vi "Panel.vi"(11 "SequenceViewPanel in":refnum<class "SequenceViewPanel.lvclass">) -> ()   [LabVIEW 2020, in "TSnax UI.lvlib" / "SequenceViewPanel.lvclass"]
uses:
  SequenceViewPanel.lvclass
  C:/Program Files (x86)/National Instruments/LabVIEW 2020/vi.lib/IlluminatedG/IG OOPanel/OOPanel/Panel/Panel.lvclass
  <vilib>/IlluminatedG/IG OOPanel/OOPanel/Panel/Basic UI State.ctl
  <vilib>/IlluminatedG/IG OOPanel/OOPanel/Panel/Panel Events.ctl
  <vilib>/IlluminatedG/IG OOPanel/OOPanel/Panel/Visbility Event Data.ctl
  <vilib>/IlluminatedG/IG OOPanel/OOPanel/Panel/Visibility State.ctl
  <vilib>/IlluminatedG/IG OOPanel/OOPanel/Panel/Close Reason.ctl
  Incoming Events.ctl
  Set SequenceFile Request.ctl
  TSnax/SequenceFile/SequenceFile.lvclass
  C:/dev/illuminated-g/tsnax/TSnax/PropertyObject/PropertyObject.lvclass
  SequenceViewPanel.lvclass/SequenceViewPanel.ctl
  TSnax/PropertyObject/PropertyObject.lvclass/PropertyObject.ctl
  TSnax/PropertyObject/PropertyObject Ref.vi
  TSnax/PropertyObject/PropertyObject.lvclass
  <vilib>/IlluminatedG/IG OOPanel/OOPanel/Panel/Panel.lvclass
  <vilib>/IlluminatedG/IG OOPanel/OOPanel/OOPanel.lvlib
  C:/dev/illuminated-g/tsnax/TSnax UI/SequenceViewPanel/SequenceViewPanel.lvclass
  Set SequenceFile Response.ctl
  C:/dev/illuminated-g/tsnax/TSnax/PropertyObjectFile/PropertyObjectFile.lvclass
  C:/dev/illuminated-g/tsnax/TSnax/SequenceFile/SequenceFile.lvclass
panel:
  out "Markers":picture
  in  "Steps":string(tree)
  in  "Sequences":string(tree)
  in  "Variables":string(tree)
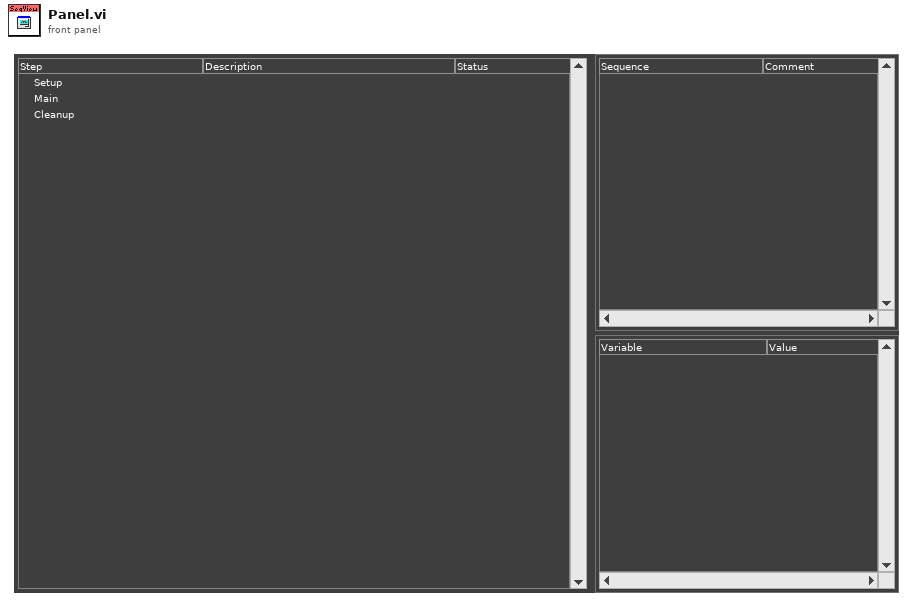
[diagram p1: front panel]
types:
  T1 = typedef "OOPanel.lvlib/Panel.lvclass/Basic UI State.ctl" = enum16{"Init", "Run", "Close"}
  T2 = typedef "TSnax UI.lvlib/SequenceViewPanel.lvclass/Set SequenceFile Response.ctl" = cluster{"Error":errorcluster}
  T3 = typedef "TSnax UI.lvlib/SequenceViewPanel.lvclass/Incoming Events.ctl" = cluster{"Set SequenceFile":refnum<user-event>}
  T4 = typedef "OOPanel.lvlib/Panel.lvclass/Panel Events.ctl" = cluster{"Visbility":refnum<user-event>, "Close":refnum<user-event>}
  T5 = cluster{"Panel":refnum<event-registration>, "Refresh Markers Reg":refnum<event-registration>}
  T6 = typedef "OOPanel.lvlib/Visibility State.ctl" = enum16{"Idle", "Closed", "Hidden", "Visible", "Subpanel"}
  T7 = typedef "LVRectTypeDef.ctl" = cluster{"Left":i16, "Top":i16, "Right":i16, "Bottom":i16}
  T8 = typedef "LVBoundsTypeDef.ctl" = cluster{"Width":u32, "Height":u32}
  T9 = typedef "LVPoint32TypeDef.ctl" = cluster{"Horizontal":i32, "Vertical":i32}
  T10 = typedef "TSnax UI.lvlib/SequenceViewPanel.lvclass/Ref Data.ctl" = cluster{"Insert Index":i32, "SequenceFile":refnum<class "SequenceFile.lvclass">}
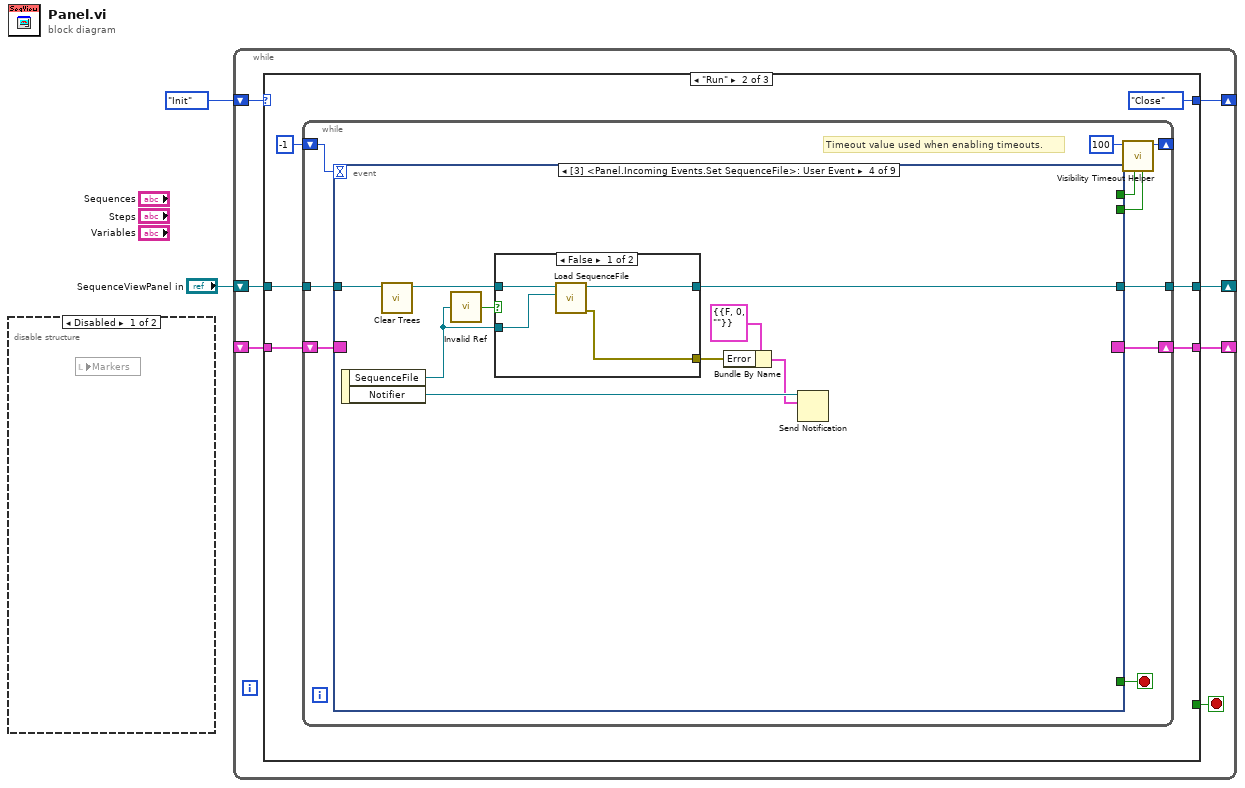
[diagram p0: block diagram]
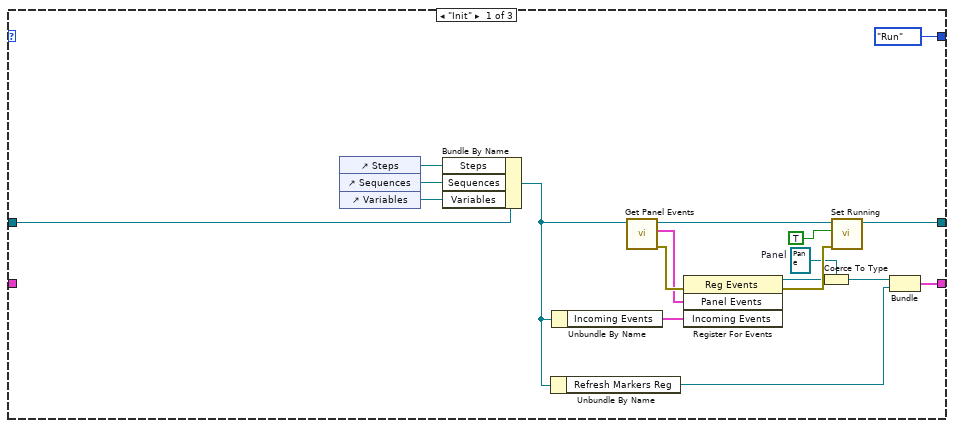
[diagram p3: hidden frame]
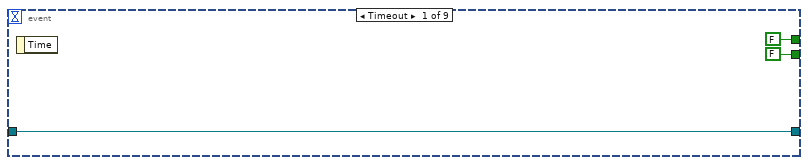
[diagram p4: hidden frame]
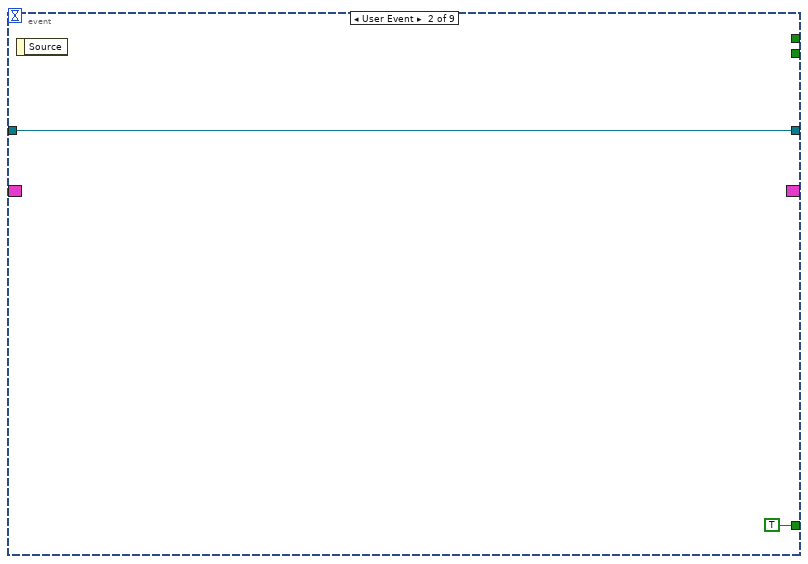
[diagram p5: hidden frame]
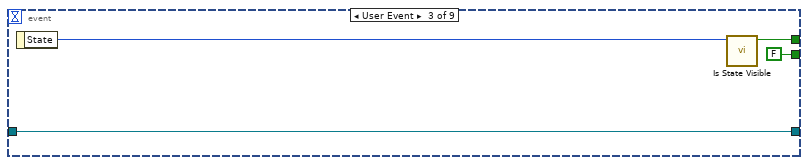
[diagram p6: hidden frame]
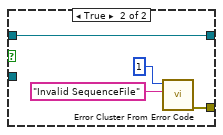
[diagram p7: hidden frame]
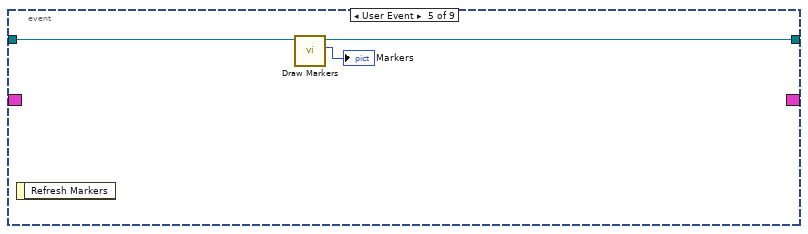
[diagram p8: hidden frame]
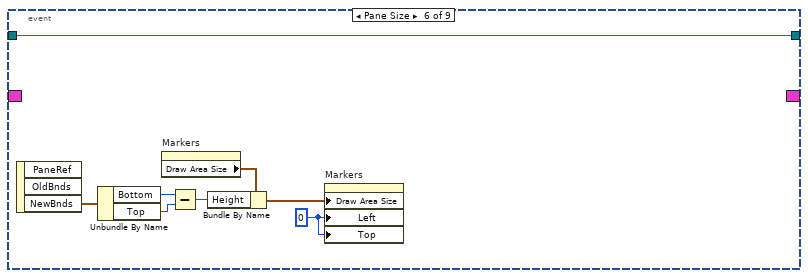
[diagram p9: hidden frame]
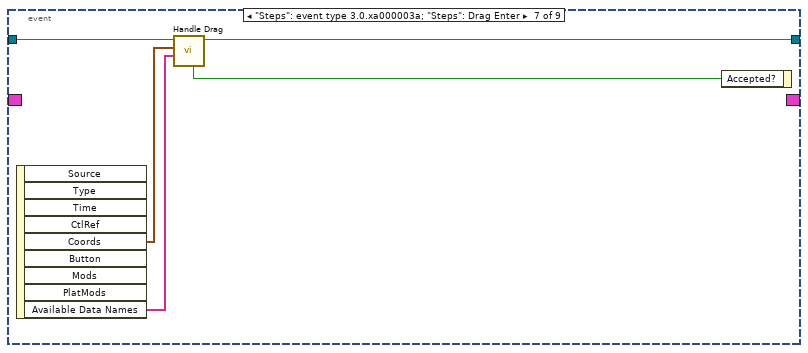
[diagram p10: hidden frame]
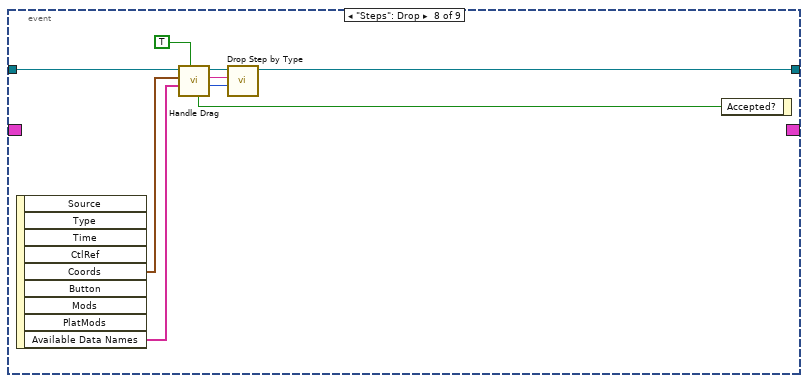
[diagram p11: hidden frame]
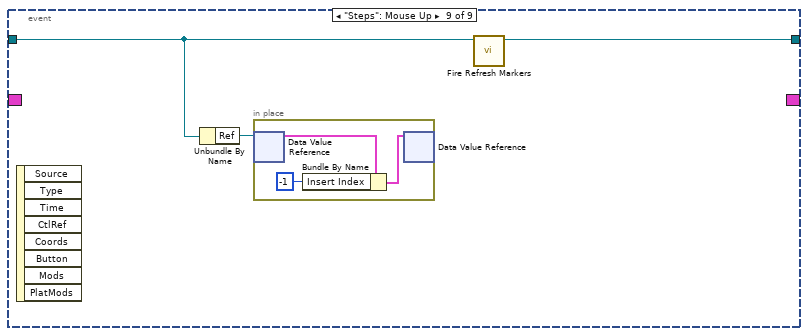
[diagram p12: hidden frame]
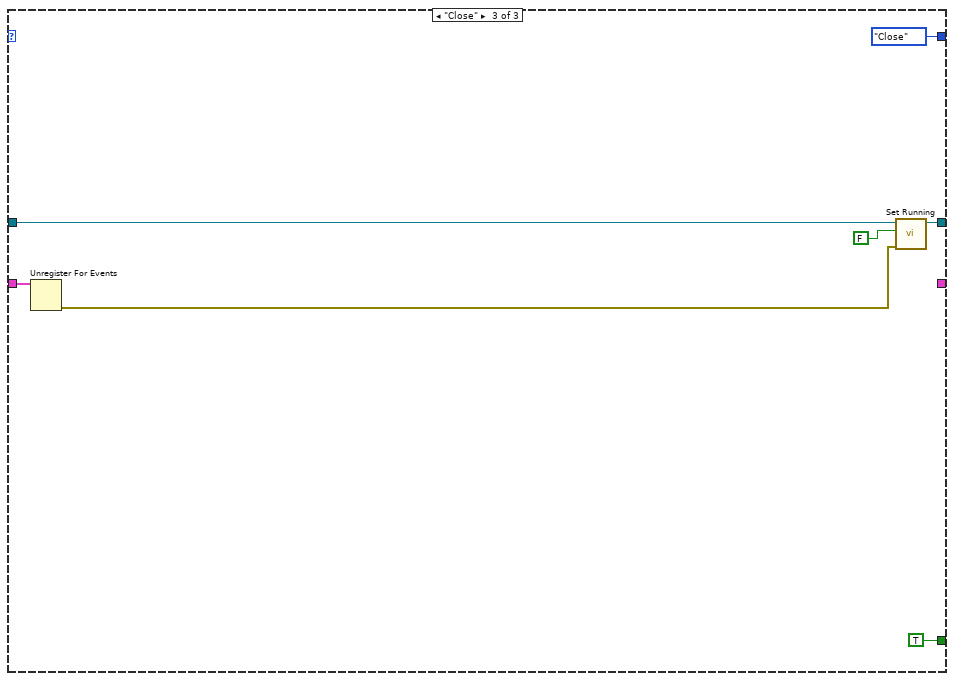
[diagram p13: hidden frame]
diagram:
  n1 = disable-structure shown="Disabled" {
    frame Disabled {
      n2 = local read "Markers"() -> ()  [unwired: 1 in]
    }
    frame Enabled {
    }
  }
  n3 = while {
    shift-right: [w8] -> _
    shift-left: _ -> [w9]
    shift-right: [w6] -> _
    shift-left: Basic_UI_State."Init" ("Basic UI State") -> [w7]
    shift-right: [w4] -> _
    shift-left: "SequenceViewPanel in" -> [w3]
    stop <- w5 stop-if-true
    n4 = case shown="\"Run\"" w7 {
      tunnel: w9 -> [_ w33 w103]
      tunnel: [w12 w31 _] -> w8
      tunnel: [Basic_UI_State."Run" ("Basic UI State") Basic_UI_State."Close" ("Basic UI State") Basic_UI_State."Close" ("Basic UI State")] -> w6
      tunnel: [_ _ TRUE] -> w5
      tunnel: [w22 w28 w101] -> w4
      tunnel: w3 -> [w17 w29 w102]
      frame "Init" {
        w10 = refnum<event-registration> refnum  # Panel
        n5 = control-ref of="Steps"() -> (w20:refnum<vi>)
        n6 = control-ref of="Sequences"() -> (w19:refnum<vi>)
        n7 = control-ref of="Variables"() -> (w18:refnum<vi>)
        n8 = Bundle By Name(cluster=w17, "Steps"=w20, "Sequences"=w19, "Variables"=w18) -> (w14:refnum<class "SequenceViewPanel.lvclass">)
        n9 = Unbundle By Name(w14) -> ("Refresh Markers Reg"=w13:refnum<event-registration>)
        n10 = Unbundle By Name(w14) -> ("Incoming Events"=w21:T3)
        n11 = call <vilib>:"Get Panel Events.vi"("Panel in"=w14) -> ("error out"=w27:errorcluster, "Panel Events"=w24:T4, "Panel out"=w16:refnum<class "SequenceViewPanel.lvclass">)  [unwired: 8 in]
        n12 = register-events(error in=w27, w24, w21) -> (reference out=w15:refnum<event-registration>, error out=w25:errorcluster)  [unwired: 1 in]
        n13 = Coerce To Type(0:w15, 1:w10) -> (2:w11:refnum<event-registration>)
        n14 = call <vilib>:"Set Running.vi"("error in (no error)"=w25, "Running"=TRUE, "Panel in"=w16) -> ("Panel out"=w22:refnum<class "SequenceViewPanel.lvclass">)  [unwired: 7 in, 1 out]
        n15 = Bundle("Panel"=w11, "Refresh Markers Reg"=w13) -> (w12:T5)  [unwired: 1 in]
      }
      frame "Run" {
        n16 = while {
          shift-right: [w39] -> w31
          shift-left: w33 -> [w40]
          shift-right: [w42] -> _
          shift-left: -1 ("Timeout") -> [w41]
          tunnel: w29 -> [w35]
          tunnel: [w34] -> w28
          stop <- w36 stop-if-true
          # "Timeout value used when enabling timeouts."
          n17 = event shown="[3] <Panel.Incoming Events.Set SequenceFile>: User Event" {
            selector: w40 -> [_ _ _ _ _ _ _ _ _]
            dyn-events: [_ _ _ _ _ _ _ _ _] -> w39
            timeout: w41 -> [_ _ _ _ _ _ _ _ _]
            tunnel: [FALSE _ w51 _ _ _ _ _ _] -> w38
            tunnel: [FALSE _ FALSE _ _ _ _ _ _] -> w37
            tunnel: [_ TRUE _ _ _ _ _ _ _] -> w36
            tunnel: w35 -> [w44 w47 w49 w61 w72 w80 w85 w94 w96]
            tunnel: [w44 w47 w49 w58 w71 w80 w82 w86 w95] -> w34
            event Timeout {
              n18 = event-data() -> ()  [unwired: 1 in, 1 out]
            }
            event User Event {
              n19 = event-data() -> ()  [unwired: 1 in, 1 out]
            }
            event User Event {
              n20 = event-data() -> ("State"=w52:T6)  [unwired: 1 in]
              n21 = call <vilib>:"Is State Visible.vi"("Visibility"=w52) -> ("Visible"=w51:bool)  [unwired: 10 in]
            }
            event User Event {
              n22 = event-data() -> ("SequenceFile"=w57:refnum<class "SequenceFile.lvclass">, "Notifier"=w56:refnum<notifier>)  [unwired: 1 in]
              n23 = call "Clear Trees.vi"("SequenceViewPanel in"=w61) -> ("SequenceViewPanel out"=w59:refnum<class "SequenceViewPanel.lvclass">)  [unwired: 9 in, 1 out]
              n24 = call "Invalid Ref.vi"("PropertyObject"=w57) -> ("Not a Valid Ref?"=w60:bool)
              n25 = case shown="False" w60 {
                tunnel: w59 -> [w65 w69]
                tunnel: [w63 w69] -> w58
                tunnel: w57 -> [w64 _]
                tunnel: [w62 w66] -> w53
                frame False {
                  n26 = call "Load SequenceFile.vi"("SequenceFile"=w64, "SequenceViewPanel in"=w65) -> ("error out"=w62:errorcluster, "SequenceViewPanel out"=w63:refnum<class "SequenceViewPanel.lvclass">)  [unwired: 8 in]
                }
                frame True {
                  n27 = call <vilib>:"Error Cluster From Error Code.vi"("error message (\"\")"="Invalid SequenceFile" ("error message (\"\")"), "error code (0)"=1) -> ("error out"=w66:errorcluster)  [unwired: 7 in]
                }
              }
              n28 = Bundle By Name(cluster=T2 {"Error"={"status"=FALSE, "code"=0, "source"=""}} ("notification"), "Error"=w53) -> (w54:T2)
              n29 = Send Notification(notification=w54, notifier=w56) -> ()  [unwired: 1 in, 2 out]
            }
            event User Event {
              n30 = event-data() -> ()  [unwired: 1 in, 1 out]
              n31 = call "Draw Markers.vi"("SequenceViewPanel in"=w72) -> ("Markers"=→"Markers":picture, "SequenceViewPanel out"=w71:refnum<class "SequenceViewPanel.lvclass">)  [unwired: 8 in, 1 out]
            }
            event Pane Size {
              w73 = 0 ("Position:Left")
              n32 = event-data() -> ("NewBnds"=w77:T7)  [unwired: 1 in, 2 out]
              n33 = Unbundle By Name(w77) -> ("Bottom"=w76:i16, "Top"=w75:i16)
              n34 = property on="Markers" class="Pict"() -> ("Draw Area Size"=w78:T8)  [unwired: 2 in, 2 out]
              n35 = Subtract(x=w76, y=w75) -> (x-y=w74:i16)
              n36 = Bundle By Name(cluster=w78, "Height"=w74) -> (w79:T8)
              n37 = property on="Markers" class="Pict"("Draw Area Size"=w79, "Left"=w73, "Top"=w73) -> ()  [unwired: 2 in, 2 out]
            }
            event "Steps": event type 3.0.xa000003a; "Steps": Drag Enter {
              n38 = event-data() -> ("Coords"=w84:T9, "Available Data Names"=w83:string[])  [unwired: 1 in, 7 out]
              n39 = call "Handle Drag.vi"("Available Data Names"=w83, "Coords"=w84, "SequenceViewPanel in"=w85) -> ("SequenceViewPanel out"=w82:refnum<class "SequenceViewPanel.lvclass">, "Accepted?"=w81:bool)  [unwired: 5 in, 2 out]
              n40 = event-data("Accepted?"=w81) -> ()  [unwired: 1 in, 1 out]
            }
            event "Steps": Drop {
              n41 = event-data() -> ("Coords"=w92:T9, "Available Data Names"=w91:string[])  [unwired: 1 in, 7 out]
              n42 = call "Handle Drag.vi"("Done? (F)"=TRUE, "Available Data Names"=w91, "Coords"=w92, "SequenceViewPanel in"=w94) -> ("Index"=w89:i32, "Step Type Name"=w87:string, "SequenceViewPanel out"=w90:refnum<class "SequenceViewPanel.lvclass">, "Accepted?"=w88:bool)  [unwired: 4 in]
              n43 = call "Drop Step by Type.vi"("Index"=w89, "Step Type Name"=w87, "SequenceViewPanel in"=w90) -> ("SequenceViewPanel out"=w86:refnum<class "SequenceViewPanel.lvclass">)  [unwired: 7 in, 1 out]
              n44 = event-data("Accepted?"=w88) -> ()  [unwired: 1 in, 1 out]
            }
            event "Steps": Mouse Up {
              n45 = event-data() -> ()  [unwired: 1 in, 8 out]
              n46 = Unbundle By Name(w96) -> ("Ref"=w97:refnum<data-value>)
              n47 = in-place {
                n48 = in-place-dvr #1(w97) -> (w100:T10)  [unwired: 1 out]
                n49 = Bundle By Name(cluster=w100, "Insert Index"=-1) -> (w99:T10)
                n50 = in-place-dvr #1(w99) -> ()  [unwired: 2 out]
              }
              n51 = call "Fire Refresh Markers.vi"("SequenceViewPanel in"=w96) -> ("SequenceViewPanel out"=w95:refnum<class "SequenceViewPanel.lvclass">)  [unwired: 9 in, 1 out]
            }
          }
          n52 = call <vilib>:"Visibility Timeout Helper.vi"("Update?"=w37, "Use Timeout?"=w38, "Visible Timeout mS"=100) -> ("Timeout"=w42:i32)  [unwired: 8 in]
        }
      }
      frame "Close" {
        n53 = Unregister For Events(event registration refnum=w103) -> (error out=w105:errorcluster)  [unwired: 1 in]
        n54 = call <vilib>:"Set Running.vi"("error in (no error)"=w105, "Running"=FALSE, "Panel in"=w102) -> ("Panel out"=w101:refnum<class "SequenceViewPanel.lvclass">)  [unwired: 7 in, 1 out]
      }
    }
  }
